vi "CRYCalc zWicker Loudness.vi"(9 "Zwicker_X-axis":u16(ring) items=["Hz", "Bark"], 10 "Zwicker_spectrum":bool, 11 "Data in":T1={"Name"="", "Curve"=[], "X data"=1, "Y data"=1, "Z data"=1, "X axis"=0, "Y axis"=1, "Z axis"=1, "X unit"="Hz", "Y unit"="", "Z unit"="deg.", "X dB ref"=1.0, "Y dB ref"=1.0, "Z dB ref"=1.0, "single val"=FALSE, "protected"=FALSE, "display X"=TRUE, "display Y"=TRUE, "display Z"=TRUE, "Test Info"="", "Step No."=0, "Plot Settings"={"Color"=0, "Interpolation"=0, "Point Style"=0, "Line Style"=0, "Point Color"=0, "Line Width"=0, "Bar Plot Style"=0, "Fill To"=0}, "AutoProtect"=FALSE} {"Z data" items=["dB", "Lin"]; "X data" items=["dB", "Lin"]; "Y data" items=["dB", "Lin"]; "Z dB ref" format="%.1f"; "Z axis" items=["Log", "Lin"]; "X dB ref" format="%.1f"; "X axis" items=["Log", "Lin"]; "Y axis" items=["Log", "Lin"]; "Y dB ref" format="%.1f"; "Curve"."z" format="%.2f"; "Curve"."y" format="%.2f"; "Curve"."x" format="%.2f"}) -> (0 "z":dbl, 1 "y":dbl, 2 "x":dbl, 3 "Curve":cluster{"x":dbl, "y":dbl, "z":dbl}[](array[cluster]))   [LabVIEW 2013]
uses:
  Typedef Control/CRYData Cluster.ctl
panel:
  out "SPL 2":dbl[](array[numeric])
  out "SPL":dbl[](array[numeric])
  out "frequency":dbl[](array[numeric])
  in  "outZ":dbl[](array[numeric])
  in  "outX":dbl[](array[numeric])
  in  "outY":dbl[](array[numeric])
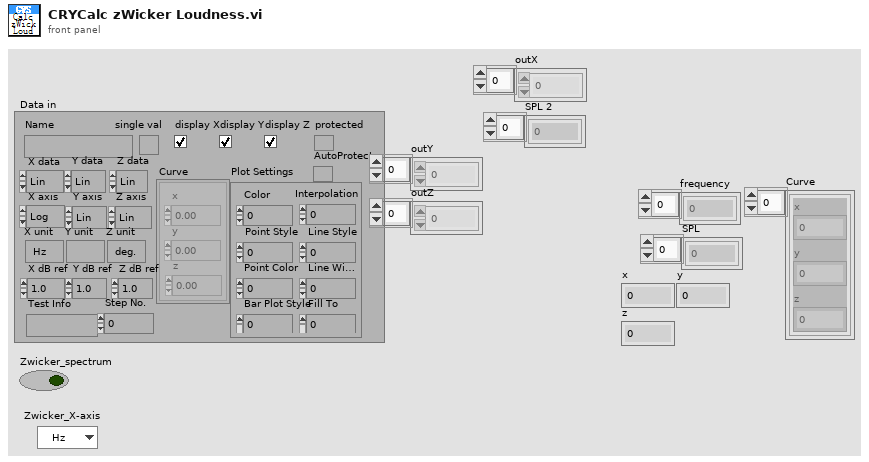
[diagram p1: front panel]
types:
  T1 = typedef "CRYData Cluster.ctl" = cluster{"Name":string, "Curve":cluster{"x":dbl, "y":dbl, "z":dbl}[], "X data":u16, "Y data":u16, "Z data":u16, "X axis":u16, "Y axis":u16, "Z axis":u16, "X unit":string, "Y unit":string, "Z unit":string, "X dB ref":dbl, "Y dB ref":dbl, "Z dB ref":dbl, "single val":bool, "protected":bool, "display X":bool, "display Y":bool, "display Z":bool, "Test Info":string, "Step No.":i32, "Plot Settings":cluster{"Color":u32, "Interpolation":u8, "Point Style":u8, "Line Style":u8, "Point Color":u32, "Line Width":u8, "Bar Plot Style":u8, "Fill To":i16}, "AutoProtect":bool}
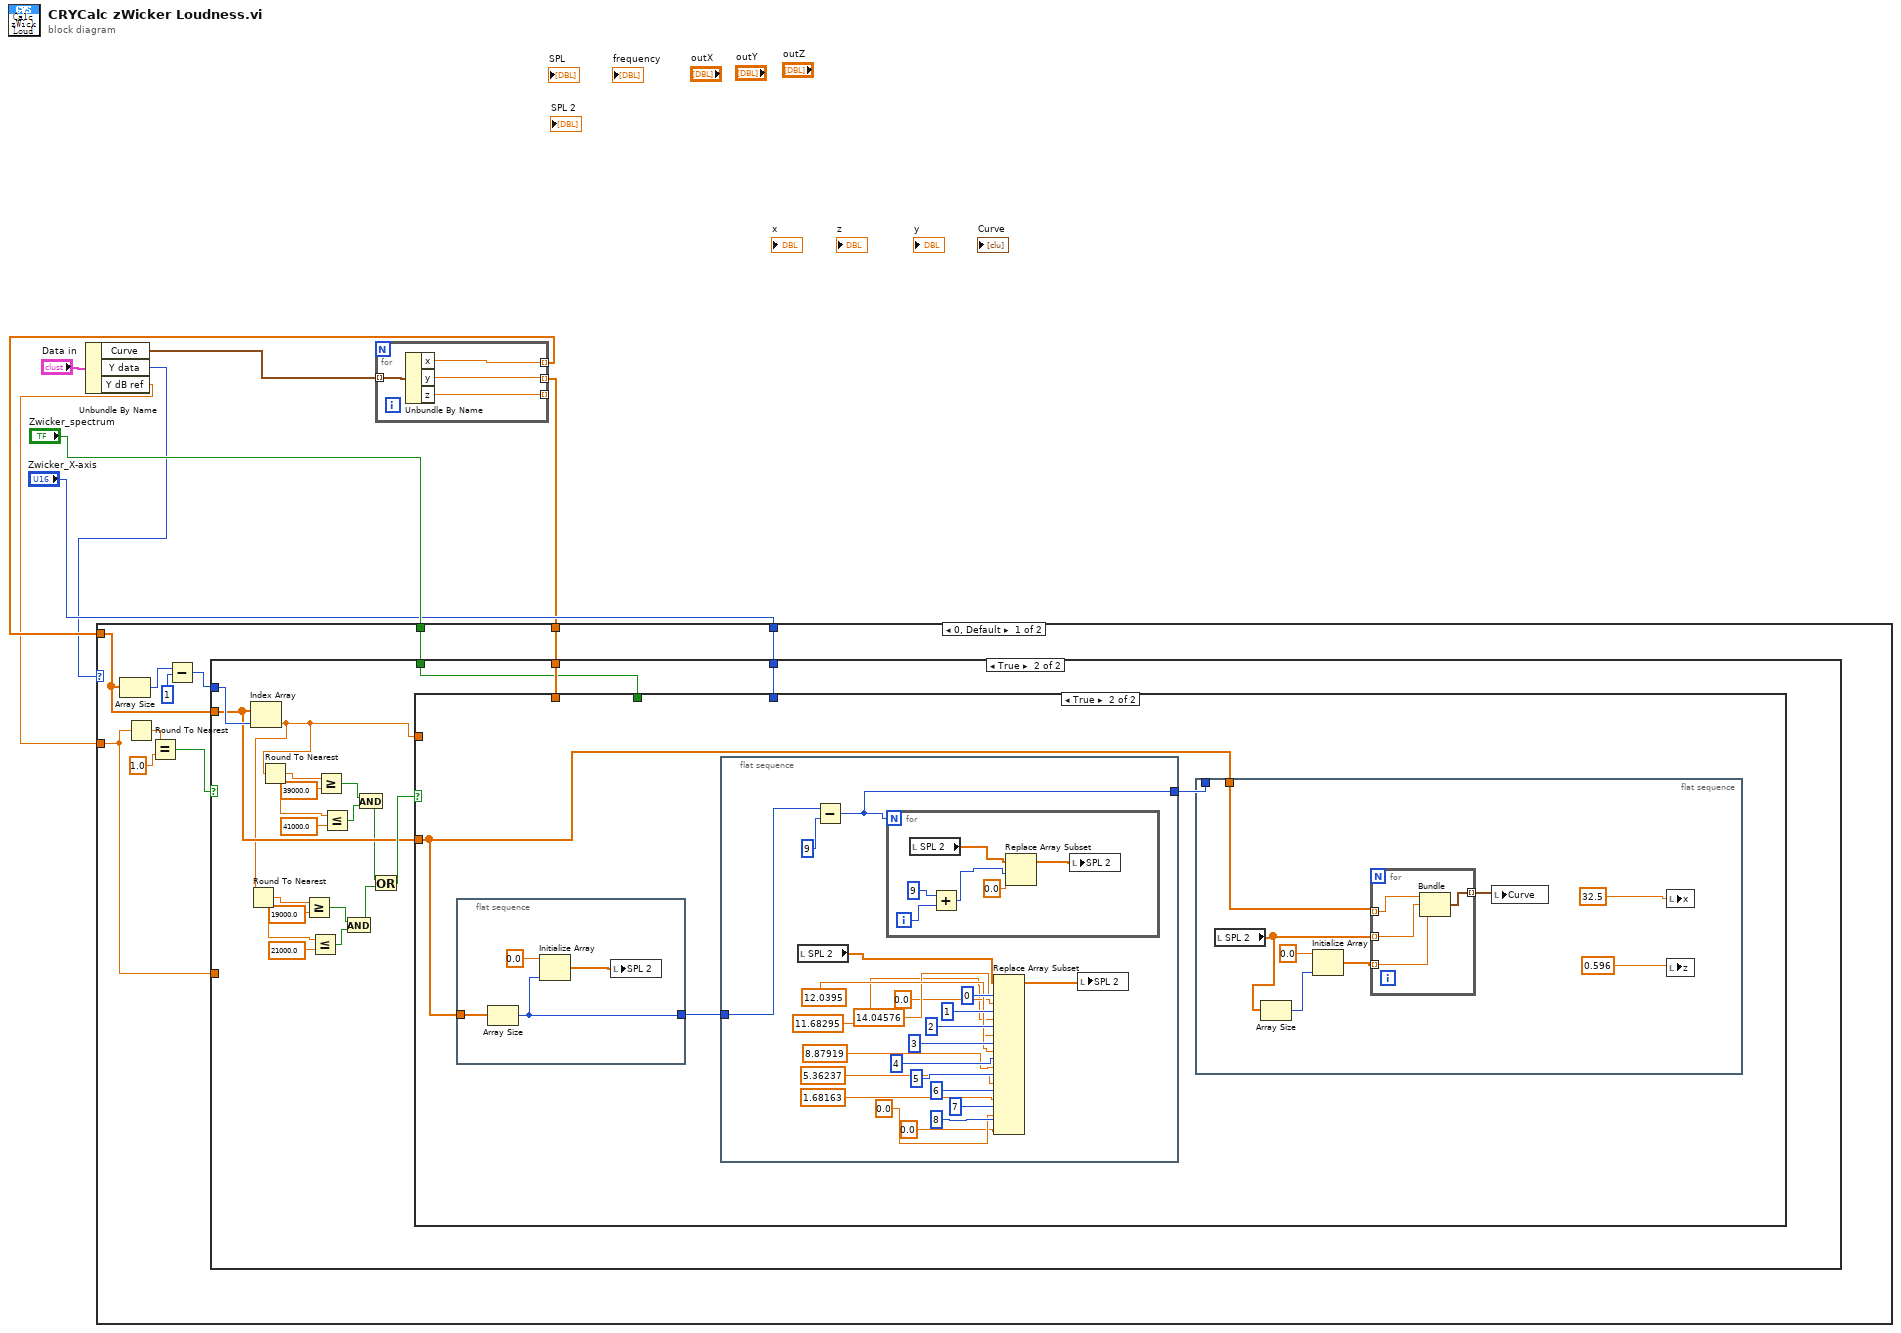
[diagram p0: block diagram]
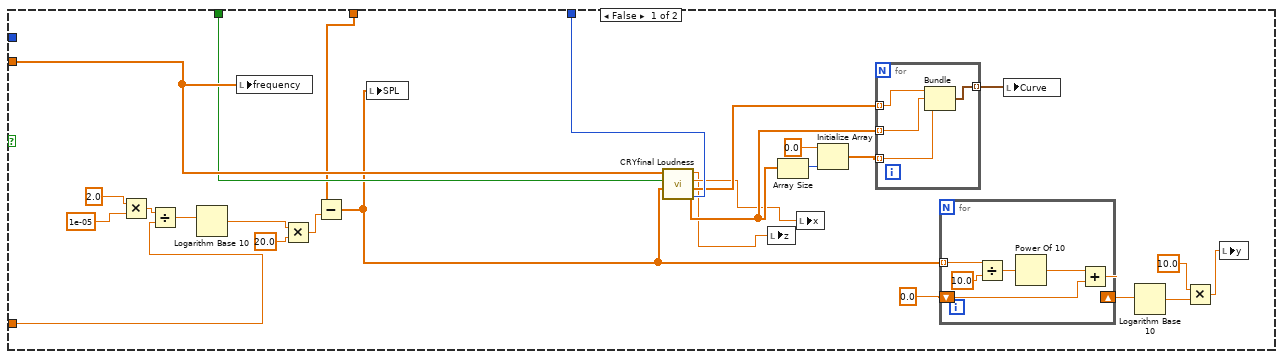
[diagram p2: hidden frame]
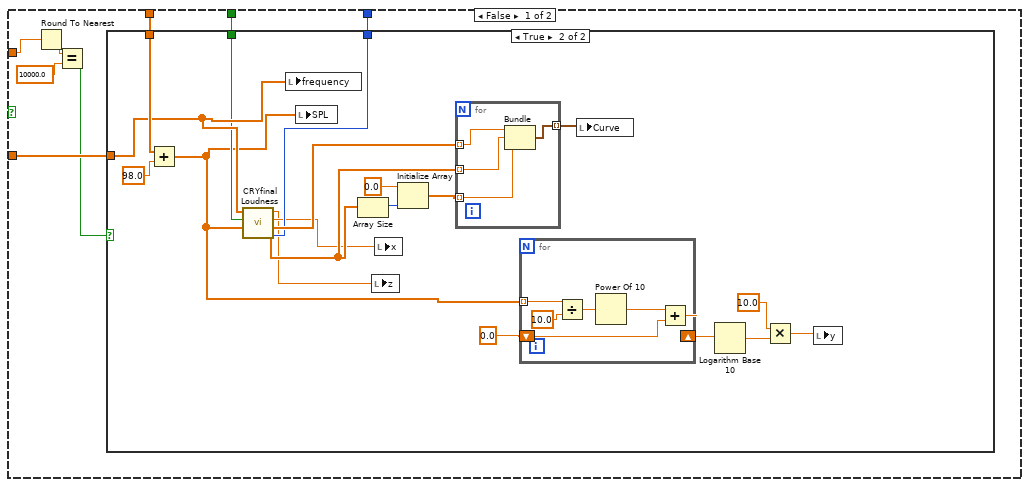
[diagram p3: hidden frame]
diagram:
  n1 = Unbundle By Name("Data in") -> ("Curve"=w7:cluster{"x":dbl, "y":dbl, "z":dbl}[], "Y data"=w1:u16, "Y dB ref"=w2:dbl)
  n2 = for {
    tunnel: w7 -> [w12] mode=indexing
    tunnel: [w11] -> w4 mode=indexing
    tunnel: [w10] -> w3 mode=indexing
    tunnel: [w9] -> _ mode=indexing
    n3 = Unbundle By Name(w12) -> ("x"=w11:dbl, "y"=w10:dbl, "z"=w9:dbl)
  }
  n4 = case shown="0, Default" w1 {
    tunnel: w2 -> [w14 _]
    tunnel: w4 -> [w22 _]
    tunnel: w3 -> [w21 _]
    tunnel: "Zwicker_spectrum" -> [w20 _]
    tunnel: "Zwicker_X-axis" -> [w19 _]
    frame 0, Default {
      n5 = Array Size(array=w22) -> (size(s)=w16:i32)
      n6 = Round To Nearest(number=w14) -> (nearest integer value=w13:dbl)
      n7 = Equal?(x=w13, y=1.0) -> (x = y?=w18:bool)
      n8 = Subtract(x=w16, y=1) -> (x-y=w17:i32)
      n9 = case shown="True" w18 {
        tunnel: w22 -> [w49 w73]
        tunnel: w17 -> [_ w78]
        tunnel: w21 -> [w25 w76]
        tunnel: w20 -> [w48 w74]
        tunnel: w19 -> [w47 w75]
        tunnel: w14 -> [w30 _]
        frame False {
          n10 = Multiply(x=2.0, y=1e-05) -> (x*y=w31:dbl)
          n11 = Divide(x=w31, y=w30) -> (x/y=w29:dbl)
          n12 = Logarithm Base 10(1:w29) -> (0:w28:dbl)
          n13 = local write "frequency"(w49) -> ()
          n14 = Multiply(x=w28, y=20.0) -> (x*y=w26:dbl)
          n15 = Subtract(x=w25, y=w26) -> (x-y=w24:dbl[])
          n16 = local write "SPL"(w24) -> ()
          n17 = call "CRYfinal Loudness.vi"("Zwicker_X-axis"=w47, "SPL"=w24, "Boolean"=w48, "frequence"=w49) -> ("out Y"=w46:dbl[], "out X"=w45:dbl[], "Loud-phon"=w37:dbl, "*N(sone)"=w36:dbl)  [unwired: 4 in]
          n18 = local write "z"(w36) -> ()
          n19 = Array Size(array=w46) -> (size(s)=w38:i32)
          n20 = local write "x"(w37) -> ()
          n21 = Initialize Array(0.0, w38) -> (w40:dbl[])
          n22 = for {
            tunnel: w45 -> [w59] mode=indexing
            tunnel: w46 -> [w58] mode=indexing
            tunnel: w40 -> [w57] mode=indexing
            tunnel: [w56] -> w34 mode=indexing
            n23 = Bundle(w59, w58, w57) -> (w56:cluster{dbl, dbl, dbl})  [unwired: 1 in]
          }
          n24 = for {
            tunnel: w24 -> [w55] mode=indexing
            shift-right: [w51] -> w42
            shift-left: 0.0 -> [w50]
            n25 = Divide(x=w55, y=10.0) -> (x/y=w53:dbl)
            n26 = Power Of 10(x=w53) -> (10^x=w52:dbl)
            n27 = Add(x=w52, y=w50) -> (x+y=w51:dbl)
          }
          n28 = local write "Curve"(w34) -> ()
          n29 = Logarithm Base 10(1:w42) -> (0:w43:dbl)
          n30 = Multiply(x=10.0, y=w43) -> (x*y=w35:dbl)
          n31 = local write "y"(w35) -> ()
        }
        frame True {
          n32 = Index Array(array=w73, index=w78) -> (element=w62:dbl)
          n33 = Round To Nearest(number=w62) -> (nearest integer value=w68:dbl)
          n34 = Round To Nearest(number=w62) -> (nearest integer value=w67:dbl)
          n35 = Greater Or Equal?(x=w68, y=19000.0) -> (x >= y?=w69:bool)
          n36 = Less Or Equal?(x=w68, y=21000.0) -> (x <= y?=w70:bool)
          n37 = Greater Or Equal?(x=w67, y=39000.0) -> (x >= y?=w66:bool)
          n38 = Less Or Equal?(x=w67, y=41000.0) -> (x <= y?=w65:bool)
          n39 = And(x=w69, y=w70) -> (x .and. y?=w60:bool)
          n40 = And(x=w66, y=w65) -> (x .and. y?=w61:bool)
          n41 = Or(x=w61, y=w60) -> (x .or. y?=w77:bool)
          n42 = case shown="True" w77 {
            tunnel: w62 -> [w80 _]
            tunnel: w73 -> [w85 w117]
            tunnel: w76 -> [w83 _]
            tunnel: w75 -> [w82 _]
            tunnel: w74 -> [w81 _]
            frame False {
              n43 = Round To Nearest(number=w80) -> (nearest integer value=w79:dbl)
              n44 = Equal?(x=w79, y=10000.0) -> (x = y?=w84:bool)
              n45 = case shown="True" w84 {
                tunnel: w85 -> [_ w93]
                tunnel: w83 -> [_ w94]
                tunnel: w82 -> [_ w92]
                tunnel: w81 -> [_ w91]
                frame False {
                }
                frame True {
                  n46 = Add(x=w94, y=98.0) -> (x+y=w90:dbl[])
                  n47 = call "CRYfinal Loudness.vi"("Zwicker_X-axis"=w92, "SPL"=w90, "Boolean"=w91, "frequence"=w93) -> ("out Y"=w103:dbl[], "out X"=w102:dbl[], "Loud-phon"=w89:dbl, "*N(sone)"=w88:dbl)  [unwired: 4 in]
                  n48 = local write "frequency"(w93) -> ()
                  n49 = local write "SPL"(w90) -> ()
                  n50 = Array Size(array=w103) -> (size(s)=w95:i32)
                  n51 = local write "z"(w88) -> ()
                  n52 = local write "x"(w89) -> ()
                  n53 = Initialize Array(0.0, w95) -> (w97:dbl[])
                  n54 = for {
                    tunnel: w102 -> [w115] mode=indexing
                    tunnel: w103 -> [w114] mode=indexing
                    tunnel: w97 -> [w113] mode=indexing
                    tunnel: [w112] -> w104 mode=indexing
                    n55 = Bundle(w115, w114, w113) -> (w112:cluster{dbl, dbl, dbl})  [unwired: 1 in]
                  }
                  n56 = for {
                    tunnel: w90 -> [w111] mode=indexing
                    shift-right: [w107] -> w99
                    shift-left: 0.0 -> [w106]
                    n57 = Divide(x=w111, y=10.0) -> (x/y=w109:dbl)
                    n58 = Power Of 10(x=w109) -> (10^x=w108:dbl)
                    n59 = Add(x=w108, y=w106) -> (x+y=w107:dbl)
                  }
                  n60 = local write "Curve"(w104) -> ()
                  n61 = Logarithm Base 10(1:w99) -> (0:w100:dbl)
                  n62 = Multiply(x=10.0, y=w100) -> (x*y=w87:dbl)
                  n63 = local write "y"(w87) -> ()
                }
              }
            }
            frame True {
              n64 = flat-sequence {
                tunnel: w117 -> [w121]
                tunnel: [w119] -> w116
                frame #0 {
                  n65 = Array Size(array=w121) -> (size(s)=w119:i32)
                  n66 = Initialize Array(0.0, w119) -> (w120:dbl[])
                  n67 = local write "SPL 2"(w120) -> ()
                }
              }
              n68 = flat-sequence {
                tunnel: [w136] -> w118
                tunnel: w116 -> [w135]
                frame #0 {
                  n69 = local read "SPL 2"() -> (w137:dbl[])
                  n70 = Subtract(x=w135, y=9) -> (x-y=w136:i32)
                  n71 = for {
                    N: w136 -> [_]
                    i -> [w161]
                    n72 = local read "SPL 2"() -> (w162:dbl[])
                    n73 = Add(x=9, y=w161) -> (x+y=w159:i32)
                    n74 = Replace Array Subset(array=w162, new element=0.0, index=w159) -> (w158:dbl[])
                    n75 = local write "SPL 2"(w158) -> ()
                  }
                  n76 = Replace Array Subset(array=w137, new element #1=0.0, index #1=0, new element #2=11.68295, index #2=1, new element #3=14.04576, index #3=2, new element #4=12.0395, index #4=3, new element #5=8.87919, index #5=4, new element #6=5.36237, index #6=5, new element #7=1.68163, index #7=6, new element #8=0.0, index #8=7, new element #9=0.0, index #9=8) -> (w139:dbl[])
                  n77 = local write "SPL 2"(w139) -> ()
                }
              }
              n78 = flat-sequence {
                tunnel: w118 -> [_]
                tunnel: w117 -> [w124]
                frame #0 {
                  n79 = local read "SPL 2"() -> (w123:dbl[])
                  n80 = Array Size(array=w123) -> (size(s)=w127:i32)
                  n81 = Initialize Array(0.0, w127) -> (w129:dbl[])
                  n82 = for {
                    tunnel: w124 -> [w134] mode=indexing
                    tunnel: w123 -> [w133] mode=indexing
                    tunnel: w129 -> [w132] mode=indexing
                    tunnel: [w131] -> w130 mode=indexing
                    n83 = Bundle("x"=w134, "y"=w133, w132) -> (w131:cluster{"x":dbl, "y":dbl, dbl})  [unwired: 1 in]
                  }
                  n84 = local write "Curve"(w130) -> ()
                  n85 = local write "x"(32.5) -> ()
                  n86 = local write "z"(0.596) -> ()
                }
              }
            }
          }
        }
      }
    }
    frame 1 {
    }
  }
